vi "GetInstVisaHandle.vi"(8 "error in (no error)":errorcluster, 11 "SigGen_NIRF in":refnum<class "SigGen_NIRF.lvclass">) -> (0 "error out":errorcluster, 2 "VISA resource name out":refnum<visa-resource-name>, 3 "SigGen_NIRF out":refnum<class "SigGen_NIRF.lvclass">)   [LabVIEW 2014, in "SigGen_NIRF.lvclass"]
uses:
  SigGen_NIRF.lvclass
  SigGen_NIRF.lvclass/SigGen_NIRF.ctl
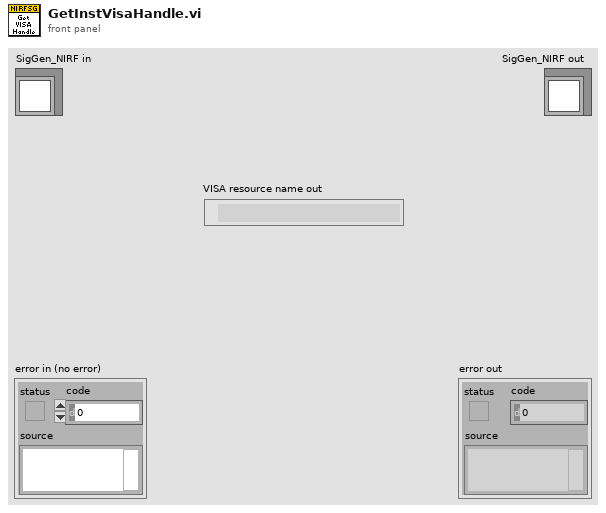
[diagram p1: front panel]
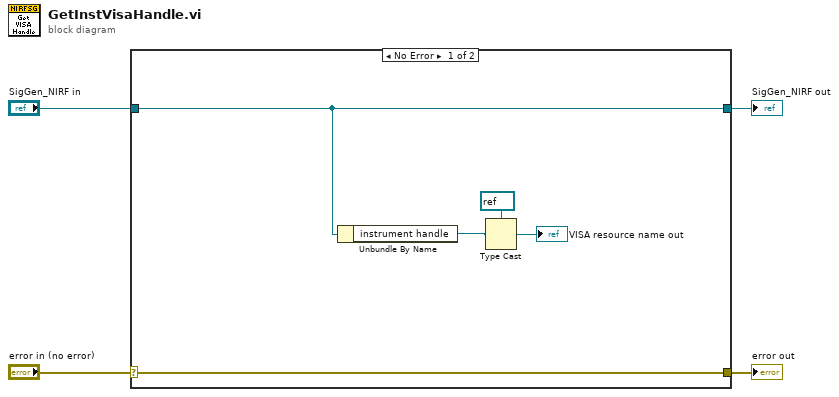
[diagram p0: block diagram]
diagram:
  n1 = case shown="No Error" "error in (no error)" {
    selector: "error in (no error)" -> [w9 w11]
    tunnel: [w9 w11] -> w3
    tunnel: [w8 w10] -> w1
    tunnel: "SigGen_NIRF in" -> [w8 w10]
    frame No Error {
      n2 = Unbundle By Name(w8) -> ("instrument handle"=w7:refnum<k15>)
      n3 = Type Cast(type=refnum<visa-resource-name> refnum ("VISA resource name out"), x=w7) -> (*(type *) &x=→"VISA resource name out":refnum<visa-resource-name>)
    }
    frame Error {
    }
  }
  "error out" <- w3
  "SigGen_NIRF out" <- w1
